vi "DependencyConstant.vi"   [LabVIEW 2020, in "OpenLvVision_OpenCv.lvlib"]
doc: "This VI makes sure the LabVIEW compile includes all necessary DLLs when you want to build an executable."
uses:
  OpenLvVision_OpenCv.lvlib
  opencv_world4130.dll
  cudnn_graph64_9.dll
  cudnn_ops64_9.dll
  Dlls/cudnn_adv64_9.dll
  cudnn64_9.dll
  Dlls/cudnn_engines_precompiled64_9.dll
  cudnn_cnn64_9.dll
  Dlls/cudnn_engines_runtime_compiled64_9.dll
  cusolver64_11.dll
  curand64_10.dll
  cufft64_11.dll
  cufftw64_11.dll
  cudart64_12.dll
  cublas64_12.dll
  nvrtc64_120_0.dll
  nvjpeg64_12.dll
  nvJitLink_120_0.dll
  cublasLt64_12.dll
  nvrtc-builtins64_129.dll
  nppig64_12.dll
  nppim64_12.dll
  nppist64_12.dll
  nppisu64_12.dll
  nppitc64_12.dll
  npps64_12.dll
  nvblas64_12.dll
  nvfatbin_120_0.dll
  nppif64_12.dll
  cusparse64_12.dll
  nppc64_12.dll
  nppial64_12.dll
  nppicc64_12.dll
  nppidei64_12.dll
  cusolverMg64_11.dll
  tbb12.dll
  Dlls/tbbbind_2_5.dll
  tbbmalloc.dll
  Dlls/tbbmalloc_proxy.dll
  openvino.dll
  Dlls/openvino_auto_batch_plugin.dll
  Dlls/openvino_auto_plugin.dll
  Dlls/openvino_c.dll
  Dlls/openvino_intel_cpu_plugin.dll
  Dlls/openvino_intel_npu_plugin.dll
  Dlls/openvino_hetero_plugin.dll
  Dlls/openvino_intel_gpu_plugin.dll
  Dlls/openvino_ir_frontend.dll
  Dlls/openvino_onnx_frontend.dll
  Dlls/openvino_paddle_frontend.dll
  Dlls/openvino_pytorch_frontend.dll
  Dlls/openvino_tensorflow_frontend.dll
  Dlls/cudnn_heuristic64_9.dll
  Dlls/OlvOpenCvWrapper.dll
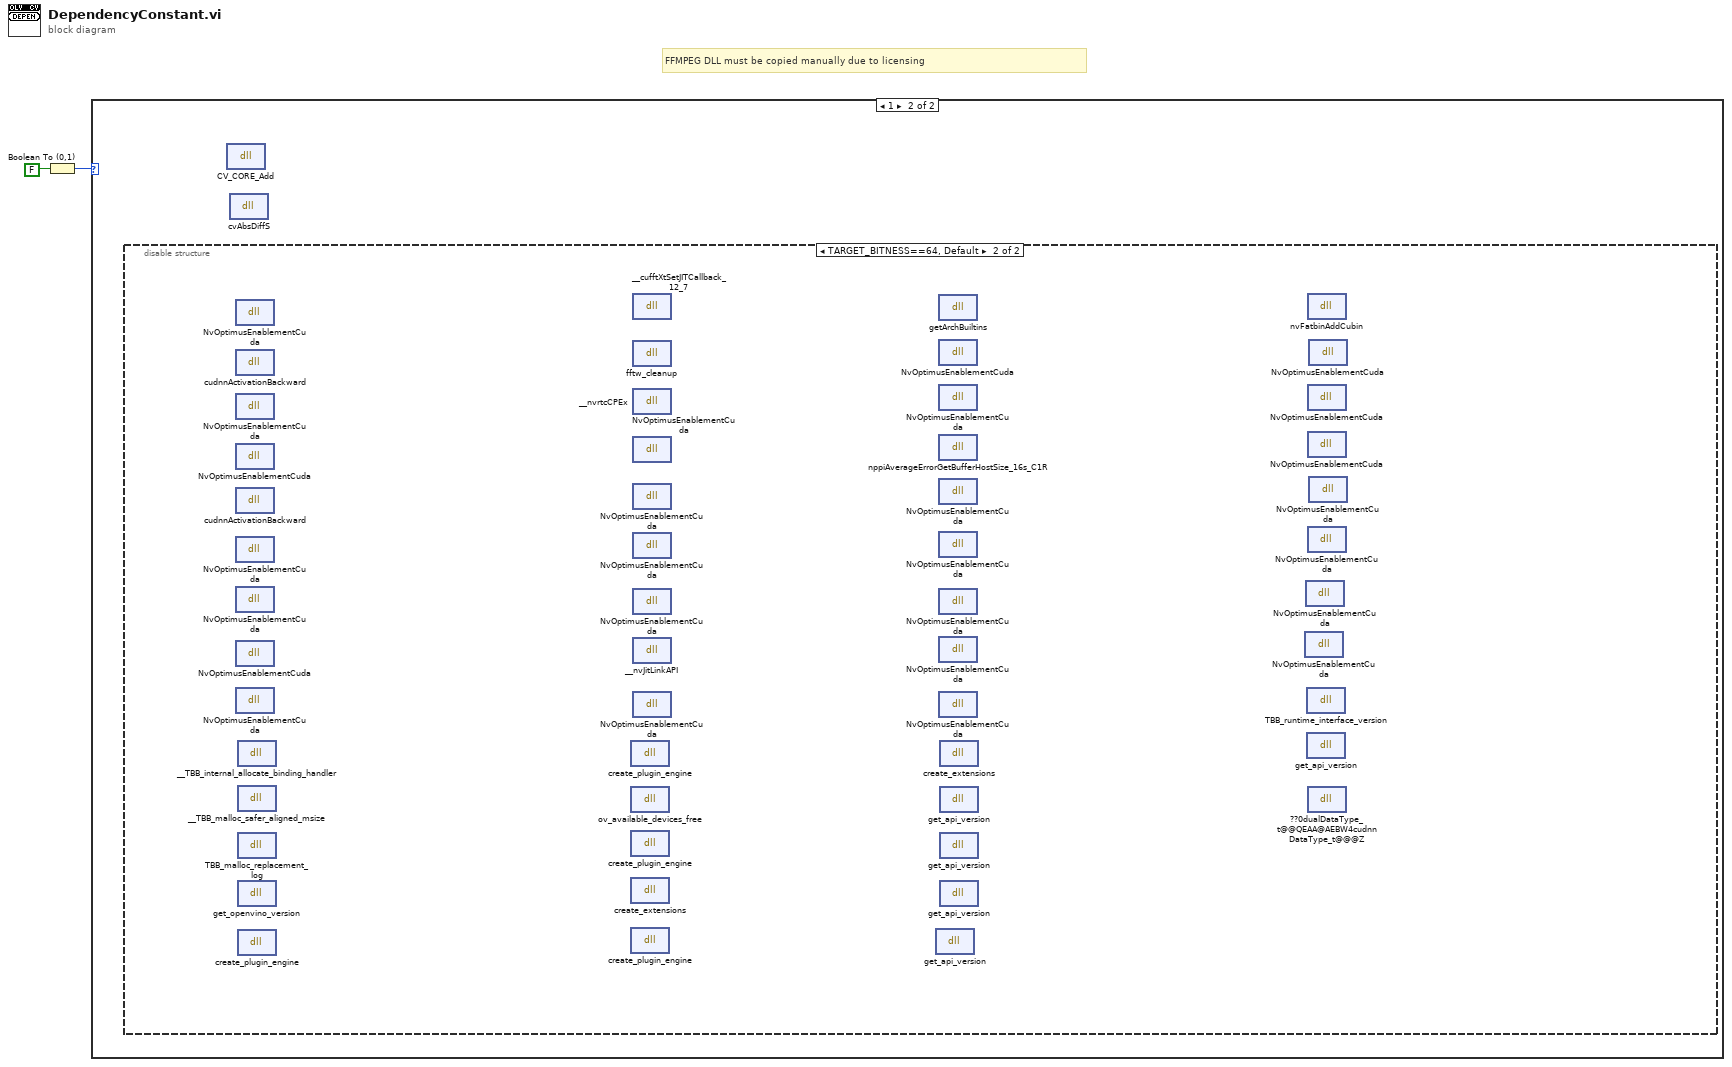
[diagram p0: block diagram]
diagram:
  # "FFMPEG DLL must be copied manually due to licensing"
  n1 = Boolean To (0,1)(Boolean=FALSE) -> (0, 1=w2:i16)
  n2 = case shown="1" w2 {
    frame 0, Default {
    }
    frame 1 {
      n3 = disable-structure shown="TARGET_BITNESS==64, Default" {
        frame condition #0 {
        }
        frame condition #1 (active) {
          n4 = dll-call lib="cudnn_graph64_9.dll" fn="NvOptimusEnablementCuda"() -> ()  [unwired: 4 in, 2 out]
          n5 = dll-call lib="cudnn_ops64_9.dll" fn="cudnnActivationBackward"() -> ()  [unwired: 4 in, 2 out]
          n6 = dll-call lib="C:/Users/lukas/Downloads/OpenLvVision_OpenCv/SourceCode/LabView/OpenLvVision_OpenCv/Dlls/cudnn_adv64_9.dll" fn="NvOptimusEnablementCuda"() -> ()  [unwired: 4 in, 2 out]
          n7 = dll-call lib="cudnn_cnn64_9.dll" fn="NvOptimusEnablementCuda"() -> ()  [unwired: 4 in, 2 out]
          n8 = dll-call lib="cudnn64_9.dll" fn="cudnnActivationBackward"() -> ()  [unwired: 4 in, 2 out]
          n9 = dll-call lib="C:/Users/lukas/Downloads/OpenLvVision_OpenCv/SourceCode/LabView/OpenLvVision_OpenCv/Dlls/cudnn_engines_precompiled64_9.dll" fn="NvOptimusEnablementCuda"() -> ()  [unwired: 4 in, 2 out]
          n10 = dll-call lib="C:/Users/lukas/Downloads/OpenLvVision_OpenCv/SourceCode/LabView/OpenLvVision_OpenCv/Dlls/cudnn_engines_runtime_compiled64_9.dll" fn="NvOptimusEnablementCuda"() -> ()  [unwired: 4 in, 2 out]
          n11 = dll-call lib="cusolver64_11.dll" fn="NvOptimusEnablementCuda"() -> ()  [unwired: 4 in, 2 out]
          n12 = dll-call lib="curand64_10.dll" fn="NvOptimusEnablementCuda"() -> ()  [unwired: 4 in, 2 out]
          n13 = dll-call lib="C:/Users/lukas/Downloads/OpenLvVision_OpenCv/SourceCode/LabView/OpenLvVision_OpenCv/Dlls/tbbbind_2_5.dll" fn="__TBB_internal_allocate_binding_handler"() -> ()  [unwired: 4 in, 2 out]
          n14 = dll-call lib="tbbmalloc.dll" fn="__TBB_malloc_safer_aligned_msize"() -> ()  [unwired: 4 in, 2 out]
          n15 = dll-call lib="C:/Users/lukas/Downloads/OpenLvVision_OpenCv/SourceCode/LabView/OpenLvVision_OpenCv/Dlls/tbbmalloc_proxy.dll" fn="TBB_malloc_replacement_log"() -> ()  [unwired: 4 in, 2 out]
          n16 = dll-call lib="openvino.dll" fn="get_openvino_version"() -> ()  [unwired: 4 in, 2 out]
          n17 = dll-call lib="C:/Users/lukas/Downloads/OpenLvVision_OpenCv/SourceCode/LabView/OpenLvVision_OpenCv/Dlls/openvino_auto_batch_plugin.dll" fn="create_plugin_engine"() -> ()  [unwired: 4 in, 2 out]
          n18 = dll-call lib="C:/Users/lukas/Downloads/OpenLvVision_OpenCv/SourceCode/LabView/OpenLvVision_OpenCv/Dlls/openvino_auto_plugin.dll" fn="create_plugin_engine"() -> ()  [unwired: 4 in, 2 out]
          n19 = dll-call lib="C:/Users/lukas/Downloads/OpenLvVision_OpenCv/SourceCode/LabView/OpenLvVision_OpenCv/Dlls/openvino_c.dll" fn="ov_available_devices_free"() -> ()  [unwired: 4 in, 2 out]
          n20 = dll-call lib="C:/Users/lukas/Downloads/OpenLvVision_OpenCv/SourceCode/LabView/OpenLvVision_OpenCv/Dlls/openvino_hetero_plugin.dll" fn="create_plugin_engine"() -> ()  [unwired: 4 in, 2 out]
          n21 = dll-call lib="C:/Users/lukas/Downloads/OpenLvVision_OpenCv/SourceCode/LabView/OpenLvVision_OpenCv/Dlls/openvino_intel_cpu_plugin.dll" fn="create_extensions"() -> ()  [unwired: 4 in, 2 out]
          n22 = dll-call lib="C:/Users/lukas/Downloads/OpenLvVision_OpenCv/SourceCode/LabView/OpenLvVision_OpenCv/Dlls/openvino_intel_gpu_plugin.dll" fn="create_plugin_engine"() -> ()  [unwired: 4 in, 2 out]
          n23 = dll-call lib="cufft64_11.dll" fn="__cufftXtSetJITCallback_12_7"() -> ()  [unwired: 4 in, 2 out]
          n24 = dll-call lib="cufftw64_11.dll" fn="fftw_cleanup"() -> ()  [unwired: 4 in, 2 out]
          n25 = dll-call lib="nvrtc64_120_0.dll" fn="__nvrtcCPEx"() -> ()  [unwired: 4 in, 2 out]
          n26 = dll-call lib="cublasLt64_12.dll" fn="NvOptimusEnablementCuda"() -> ()  [unwired: 4 in, 2 out]
          n27 = dll-call lib="cudart64_12.dll" fn="NvOptimusEnablementCuda"() -> ()  [unwired: 4 in, 2 out]
          n28 = dll-call lib="cublas64_12.dll" fn="NvOptimusEnablementCuda"() -> ()  [unwired: 4 in, 2 out]
          n29 = dll-call lib="cublas64_12.dll" fn="NvOptimusEnablementCuda"() -> ()  [unwired: 4 in, 2 out]
          n30 = dll-call lib="nvJitLink_120_0.dll" fn="__nvJitLinkAPI"() -> ()  [unwired: 4 in, 2 out]
          n31 = dll-call lib="nvjpeg64_12.dll" fn="NvOptimusEnablementCuda"() -> ()  [unwired: 4 in, 2 out]
          n32 = dll-call lib="C:/Users/lukas/Downloads/OpenLvVision_OpenCv/SourceCode/LabView/OpenLvVision_OpenCv/Dlls/openvino_pytorch_frontend.dll" fn="get_api_version"() -> ()  [unwired: 4 in, 2 out]
          n33 = dll-call lib="nvrtc-builtins64_129.dll" fn="getArchBuiltins"() -> ()  [unwired: 4 in, 2 out]
          n34 = dll-call lib="nppig64_12.dll" fn="NvOptimusEnablementCuda"() -> ()  [unwired: 4 in, 2 out]
          n35 = dll-call lib="nppim64_12.dll" fn="NvOptimusEnablementCuda"() -> ()  [unwired: 4 in, 2 out]
          n36 = dll-call lib="nppist64_12.dll" fn="nppiAverageErrorGetBufferHostSize_16s_C1R"() -> ()  [unwired: 4 in, 2 out]
          n37 = dll-call lib="nppisu64_12.dll" fn="NvOptimusEnablementCuda"() -> ()  [unwired: 4 in, 2 out]
          n38 = dll-call lib="nppitc64_12.dll" fn="NvOptimusEnablementCuda"() -> ()  [unwired: 4 in, 2 out]
          n39 = dll-call lib="nppitc64_12.dll" fn="NvOptimusEnablementCuda"() -> ()  [unwired: 4 in, 2 out]
          n40 = dll-call lib="npps64_12.dll" fn="NvOptimusEnablementCuda"() -> ()  [unwired: 4 in, 2 out]
          n41 = dll-call lib="nvblas64_12.dll" fn="NvOptimusEnablementCuda"() -> ()  [unwired: 4 in, 2 out]
          n42 = dll-call lib="C:/Users/lukas/Downloads/OpenLvVision_OpenCv/SourceCode/LabView/OpenLvVision_OpenCv/Dlls/openvino_intel_npu_plugin.dll" fn="create_extensions"() -> ()  [unwired: 4 in, 2 out]
          n43 = dll-call lib="C:/Users/lukas/Downloads/OpenLvVision_OpenCv/SourceCode/LabView/OpenLvVision_OpenCv/Dlls/openvino_ir_frontend.dll" fn="get_api_version"() -> ()  [unwired: 4 in, 2 out]
          n44 = dll-call lib="C:/Users/lukas/Downloads/OpenLvVision_OpenCv/SourceCode/LabView/OpenLvVision_OpenCv/Dlls/openvino_onnx_frontend.dll" fn="get_api_version"() -> ()  [unwired: 4 in, 2 out]
          n45 = dll-call lib="C:/Users/lukas/Downloads/OpenLvVision_OpenCv/SourceCode/LabView/OpenLvVision_OpenCv/Dlls/openvino_paddle_frontend.dll" fn="get_api_version"() -> ()  [unwired: 4 in, 2 out]
          n46 = dll-call lib="cusolverMg64_11.dll" fn="NvOptimusEnablementCuda"() -> ()  [unwired: 4 in, 2 out]
          n47 = dll-call lib="nppidei64_12.dll" fn="NvOptimusEnablementCuda"() -> ()  [unwired: 4 in, 2 out]
          n48 = dll-call lib="tbb12.dll" fn="TBB_runtime_interface_version"() -> ()  [unwired: 4 in, 2 out]
          n49 = dll-call lib="C:/Users/lukas/Downloads/OpenLvVision_OpenCv/SourceCode/LabView/OpenLvVision_OpenCv/Dlls/openvino_tensorflow_frontend.dll" fn="get_api_version"() -> ()  [unwired: 4 in, 2 out]
          n50 = dll-call lib="nvfatbin_120_0.dll" fn="nvFatbinAddCubin"() -> ()  [unwired: 4 in, 2 out]
          n51 = dll-call lib="cusparse64_12.dll" fn="NvOptimusEnablementCuda"() -> ()  [unwired: 4 in, 2 out]
          n52 = dll-call lib="nppc64_12.dll" fn="NvOptimusEnablementCuda"() -> ()  [unwired: 4 in, 2 out]
          n53 = dll-call lib="nppicc64_12.dll" fn="NvOptimusEnablementCuda"() -> ()  [unwired: 4 in, 2 out]
          n54 = dll-call lib="C:/Users/lukas/Downloads/OpenLvVision_OpenCv/SourceCode/LabView/OpenLvVision_OpenCv/Dlls/cudnn_heuristic64_9.dll" fn="??0dualDataType_t@@QEAA@AEBW4cudnnDataType_t@@@Z"() -> ()  [unwired: 4 in, 2 out]
          n55 = dll-call lib="nppif64_12.dll" fn="NvOptimusEnablementCuda"() -> ()  [unwired: 4 in, 2 out]
          n56 = dll-call lib="nppial64_12.dll" fn="NvOptimusEnablementCuda"() -> ()  [unwired: 4 in, 2 out]
        }
      }
      n57 = dll-call lib="C:/Users/lukas/Downloads/OpenLvVision_OpenCv/SourceCode/LabView/OpenLvVision_OpenCv/Dlls/OlvOpenCvWrapper.dll" fn="CV_CORE_Add"() -> ()  [unwired: 4 in, 2 out]
      n58 = dll-call lib="opencv_world4130.dll" fn="cvAbsDiffS"() -> ()  [unwired: 4 in, 2 out]
    }
  }
